vi "Scale_Raw_to_EU.vi"(10 "ConfigScale":T1={"scale [EU/RAW]"=1.0, "offset [EU]"=0.0} {"offset [EU]" format="%0.2f"; "scale [EU/RAW]" format="%0.2f"}, 11 "RAW":dbl) -> (3 "EU":dbl)   [LabVIEW 2019]
uses:
  TypeDef/Config_Scale.ctl
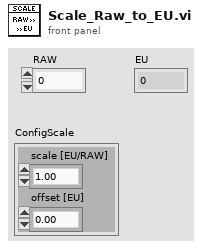
[diagram p1: front panel]
types:
  T1 = typedef "Config_Scale.ctl" = cluster{"scale [EU/RAW]":dbl, "offset [EU]":dbl}
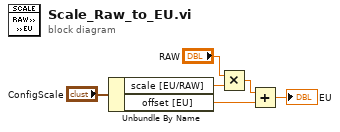
[diagram p0: block diagram]
diagram:
  n1 = Unbundle By Name("ConfigScale") -> ("scale [EU/RAW]"=w5:dbl, "offset [EU]"=w2:dbl)
  n2 = Multiply(x="RAW", y=w5) -> (x*y=w3:dbl)
  n3 = Add(x=w3, y=w2) -> (x+y=→"EU":dbl)
